vi "Flatten.vi"(8 "error in (no error)":errorcluster, 11 "Wavelength PEM and Digikröm in":refnum<class "Wavelength PEM and Digikröm.lvclass">) -> (0 "error out":errorcluster, 3 "Wavelength PEM and Digikröm out":refnum<class "Wavelength PEM and Digikröm.lvclass">)   [LabVIEW 2017, in "Wavelength PEM and Digikröm.lvclass"]
uses:
  Global/File Locations.vi
  Scanner/Scanner.lvclass
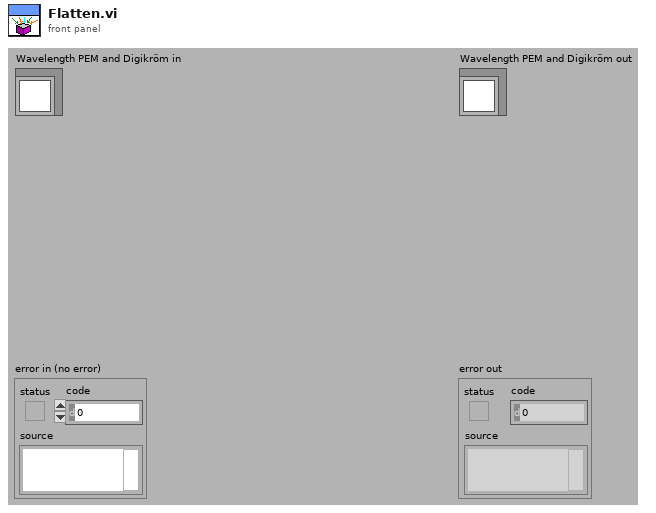
[diagram p1: front panel]
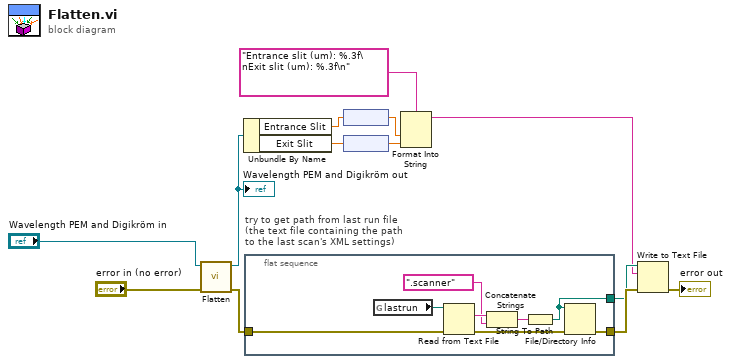
[diagram p0: block diagram]
diagram:
  n1 = call-parent "Flatten.vi"("error in (no error)"="error in (no error)", "Scanner in"="Wavelength PEM and Digikröm in") -> ("error out"=w13:errorcluster, "Scanner out"=w2:refnum<class "Wavelength PEM and Digikröm.lvclass">)  [unwired: 8 in]
  "Wavelength PEM and Digikröm out" <- w2
  n2 = Unbundle By Name(w2) -> ("Entrance Slit"=w10:dbl[unit], "Exit Slit"=w9:dbl[unit])
  n3 = flat-sequence "try to get path from last run file\n(the text file containing the path\nto the last scan's XML settings)" {
    tunnel: [w21] -> w11
    tunnel: [w18] -> w12
    tunnel: w13 -> [w17]
    frame #0 {
      n4 = global read "File Locations.vi" "lastrun"() -> (w20:path)
      n5 = Read from Text File(file (use dialog)=w20, error in=w17) -> (text=w16:string, error out=w19:errorcluster)  [unwired: 4 out]
      n6 = Concatenate Strings(w16, ".scanner") -> (w14:string)
      n7 = String To Path(string=w14) -> (path=w21:path)
      n8 = File/Directory Info(path=w21, error in=w19) -> (error out=w18:errorcluster)  [unwired: 6 out]
    }
  }
  n9 = node(w10) -> (w7:dbl)
  n10 = node(w9) -> (w5:dbl)
  n11 = Format Into String(format string="Entrance slit (um): %.3f\nExit slit (um): %.3f\n", w7, w5) -> (resulting string=w6:string)  [unwired: 2 in, 1 out]
  n12 = Write to Text File(file (use dialog)=w11, text=w6, error in=w12) -> (error out=→"error out":errorcluster)  [unwired: 1 in, 2 out]
